vi "Measure DC Volts3.vi"(10 "measurementservice_DMMConfigRequest_Data":T1, 11 "IVI Refnum in":refnum<k15>="DMM" caption="Device Name") -> (0 "error out":errorcluster, 2 "Measurement Array (Volts)":dbl[](array[numeric]))   [LabVIEW 2019, in "HVC3.lvlib" / "HVC3.lvclass"]
uses:
  HVC3 Class/HVC3.lvclass
  HVC3 Class/RPC Messages/measurementservice_DMMConfigRequest/measurementservice_DMMConfigRequest_Data.ctl
  <instrlib>/niDMM/nidmm.llb/niDMM Configure Measurement Digits.vi
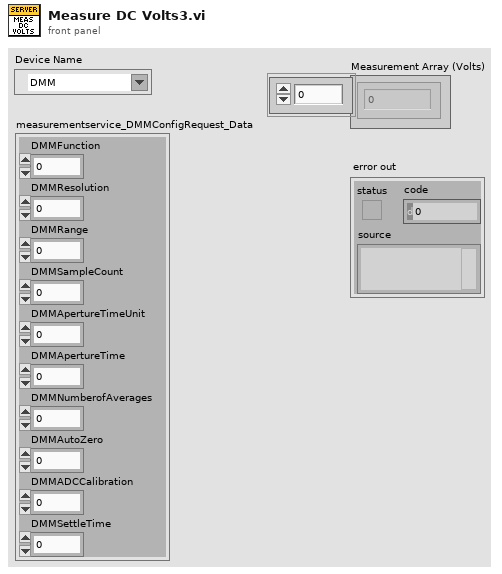
[diagram p1: front panel]
types:
  T1 = typedef "HVC3.lvlib/HVC3.lvclass/measurementservice_DMMConfigRequest_Data.ctl" = cluster{"DMMFunction":i32, "DMMResolution":sgl, "DMMRange":sgl, "DMMSampleCount":i32, "DMMApertureTimeUnit":i32, "DMMApertureTime":sgl, "DMMNumberofAverages":i32, "DMMAutoZero":i32, "DMMADCCalibration":i32, "DMMSettleTime":sgl}
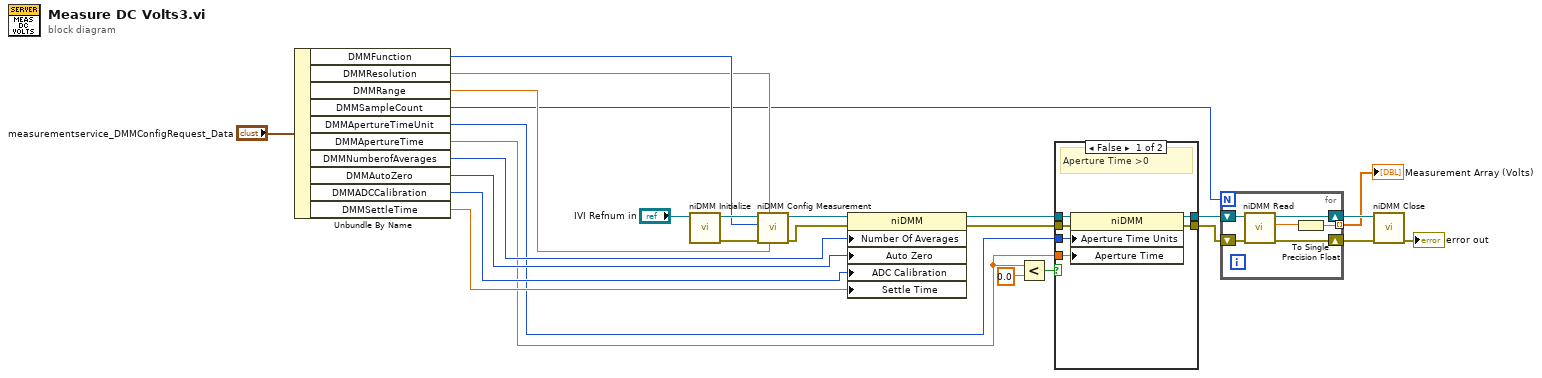
[diagram p0: block diagram]
diagram:
  n1 = Unbundle By Name("measurementservice_DMMConfigRequest_Data") -> ("DMMFunction"=w20:i32, "DMMResolution"=w19:sgl, "DMMRange"=w18:sgl, "DMMSampleCount"=w17:i32, "DMMApertureTimeUnit"=w4:i32, "DMMApertureTime"=w3:sgl, "DMMNumberofAverages"=w14:i32, "DMMAutoZero"=w13:i32, "DMMADCCalibration"=w12:i32, "DMMSettleTime"=w11:sgl)
  n2 = call <instrlib>:"niDMM Initialize.vi"("Instrument Descriptor"="IVI Refnum in") -> ("error out"=w24:errorcluster, "instrument handle out"=w25:refnum<k15>)  [unwired: 9 in]
  n3 = call-poly <instrlib>:"niDMM Config Measurement.vi"("Range"=w18, "Resolution in Digits"=w19, "error in (no error)"=w24, "Function"=w20, "instrument handle"=w25) -> ("error out"=w15:errorcluster, "instrument handle out"=w16:refnum<k15>)  [unwired: 5 in]
  n4 = property class="niDMM"(reference=w16, error in=w15, "Number Of Averages"=w14, "Auto Zero"=w13, "ADC Calibration"=w12, "Settle Time"=w11) -> (reference out=w10:refnum<k15>, error out=w9:errorcluster)
  n5 = Less?(x=w3, y=0.0 ("Configuration:Advanced:Aperture Time")) -> (x < y?=w5:bool)
  n6 = case shown="False" w5 {
    tunnel: w10 -> [w32 w34]
    tunnel: w9 -> [w31 w33]
    tunnel: [w30 w34] -> w8
    tunnel: [w29 w33] -> w7
    tunnel: w4 -> [w28 _]
    tunnel: w3 -> [w27 _]
    frame False {
      # "Aperture Time >0"
      n7 = property class="niDMM"(reference=w32, error in=w31, "Aperture Time Units"=w28, "Aperture Time"=w27) -> (reference out=w30:refnum<k15>, error out=w29:errorcluster)
    }
    frame True {
      # "Aperture Time <0"
    }
  }
  n8 = for {
    N: w17 -> [_]
    tunnel: [w35] -> w1 mode=indexing
    shift-right: [w39] -> w21
    shift-left: w7 -> [w38]
    shift-right: [w40] -> w22
    shift-left: w8 -> [w37]
    n9 = call <instrlib>:"niDMM Read.vi"("error in (no error)"=w38, "instrument handle"=w37) -> ("error out"=w39:errorcluster, "Measurement"=w36:dbl, "instrument handle out"=w40:refnum<k15>)  [unwired: 7 in]
    n10 = To Single Precision Float(number=w36) -> (single precision float=w35:sgl)
  }
  "Measurement Array (Volts)" <- w1
  n11 = call <instrlib>:"niDMM Close.vi"("error in (no error)"=w21, "instrument handle"=w22) -> ("error out"=→"error out":errorcluster)  [unwired: 9 in]
